vi "Create All Message Queues.vi"(8 "error in (no error)":errorcluster) -> (0 "error out":errorcluster, 3 "Message Queues out":T1)   [LabVIEW 2019, in "Instrument.Lockin.lvlib" / "Message Queue.lvlib"]
doc: "This VI creates and initializes all the message queues for your application. If your application requires more than one message queue, right-click the \"Message Queues\" constant above and select Open Type Def. Add the new Message Queue(s) to the type definition, then initialize them in this VI."
uses:
  Message Queue.lvlib
  All Message Queues.ctl
  Message Cluster.ctl
  Enqueue Message (Single).vi
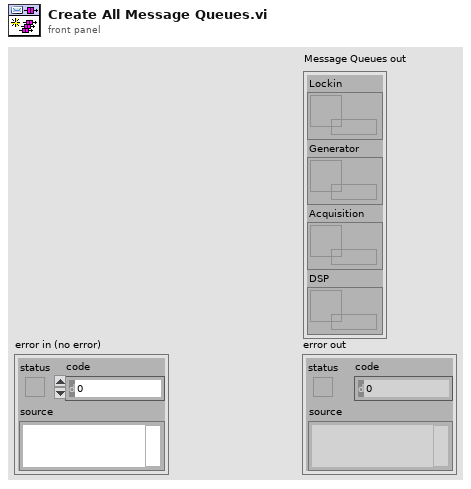
[diagram p1: front panel]
types:
  T1 = typedef "Instrument.Lockin.lvlib/Message Queue.lvlib/All Message Queues.ctl" = cluster{"Lockin":refnum<queue>, "Generator":refnum<queue>, "Acquisition":refnum<queue>, "DSP":refnum<queue>}
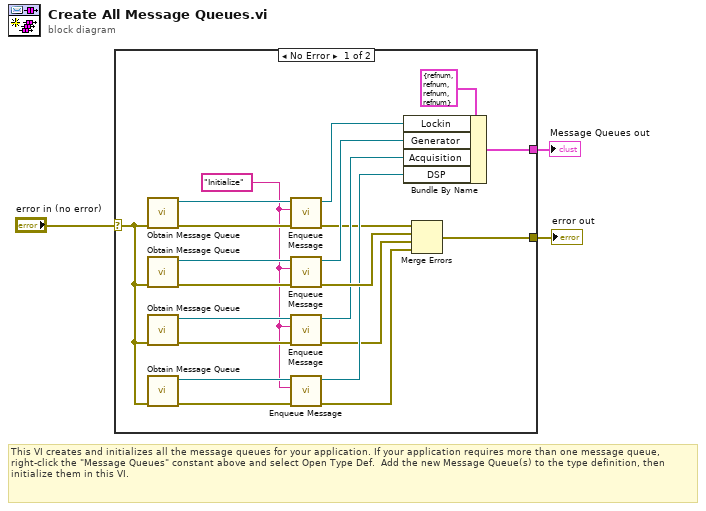
[diagram p0: block diagram]
diagram:
  # "This VI creates and initializes all the message queues for your application. If your application requires more than one message queue, right-click the \"Message Queues\" constant above and select Open Type Def.  Add the new Message Queue(s) to the type definition, then initialize them in this VI."
  n1 = case shown="No Error" "error in (no error)" {
    selector: "error in (no error)" -> [w5 w25]
    tunnel: [w13 w25] -> w3
    tunnel: [w23 _] -> w2
    frame No Error {
      w4 = "Initialize" ("Message")
      n2 = call "Obtain Message Queue.vi"("error in (no error)"=w5) -> ("error out"=w6:errorcluster, "Message Queue"=w9:refnum<queue>)  [unwired: 9 in]
      n3 = call "Obtain Message Queue.vi"("error in (no error)"=w5) -> ("error out"=w22:errorcluster, "Message Queue"=w21:refnum<queue>)  [unwired: 9 in]
      n4 = call "Obtain Message Queue.vi"("error in (no error)"=w5) -> ("error out"=w19:errorcluster, "Message Queue"=w20:refnum<queue>)  [unwired: 9 in]
      n5 = call "Obtain Message Queue.vi"("error in (no error)"=w5) -> ("error out"=w18:errorcluster, "Message Queue"=w17:refnum<queue>)  [unwired: 9 in]
      n6 = call-poly "Enqueue Message.vi"("error in (no error)"=w6, "Message"=w4, "Message Queue"=w9) -> ("error out"=w7:errorcluster, "dup Message Queue"=w8:refnum<queue>)  [unwired: 7 in]
      n7 = call-poly "Enqueue Message.vi"("error in (no error)"=w22, "Message"=w4, "Message Queue"=w21) -> ("error out"=w24:errorcluster, "dup Message Queue"=w16:refnum<queue>)  [unwired: 7 in]
      n8 = call-poly "Enqueue Message.vi"("error in (no error)"=w19, "Message"=w4, "Message Queue"=w20) -> ("error out"=w12:errorcluster, "dup Message Queue"=w15:refnum<queue>)  [unwired: 7 in]
      n9 = call-poly "Enqueue Message.vi"("error in (no error)"=w18, "Message"=w4, "Message Queue"=w17) -> ("error out"=w11:errorcluster, "dup Message Queue"=w14:refnum<queue>)  [unwired: 7 in]
      n10 = Bundle By Name(cluster=T1 {"Lockin"=refnum, "Generator"=refnum, "Acquisition"=refnum, "DSP"=refnum} ("Message Queues"), "Lockin"=w8, "Generator"=w16, "Acquisition"=w15, "DSP"=w14) -> (w23:T1)
      n11 = Merge Errors(w7, w24, w12, w11) -> (w13:errorcluster)
    }
    frame Error {
    }
  }
  "Message Queues out" <- w2
  "error out" <- w3
